vi "db_link.vi"(2 "Current time":timestamp, 4 "SaveNow":bool, 6 "Continuosly":bool, 7 "SaveCurves?":bool, 8 "error in":errorcluster, 9 "AllMeasures":cluster{"x0":dbl, "dx":dbl, "y":sgl[][]}[](array[cluster]), 10 "Table":string[][](array[string]), 11 "reference":refnum<vi>) -> (0 "error":errorcluster)   [LabVIEW 2010]
uses:
  70user.lib/TheSigTab.vi
  <vilib>/addons/database/NI_Database_API.lvlib
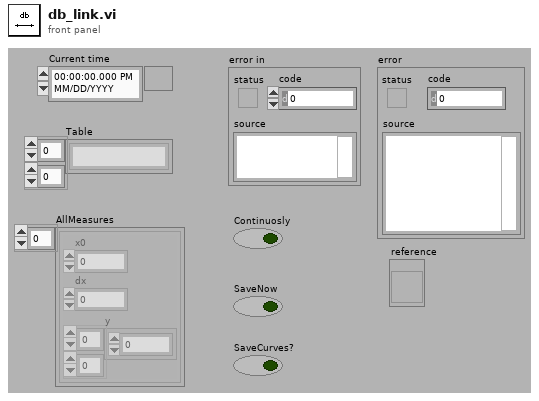
[diagram p1: front panel]
types:
  T1 = typedef "NI_Database_API.lvlib/Conn ObjectReference.ctl" = refnum<k1>
  T2 = cluster{"date/time string":string, "Reason 2":string}
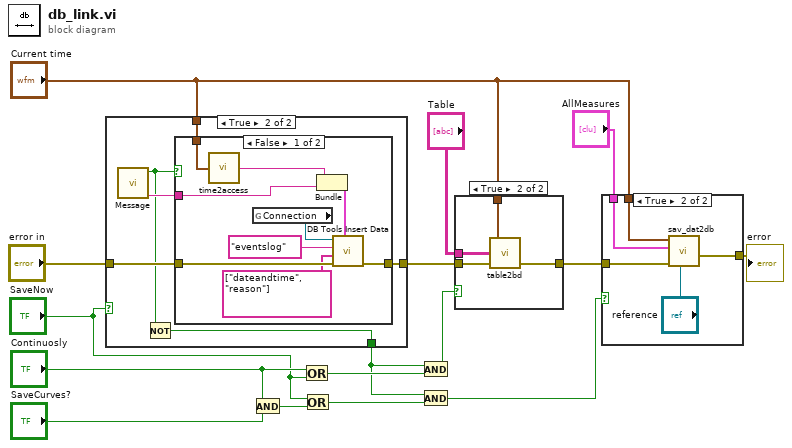
[diagram p0: block diagram]
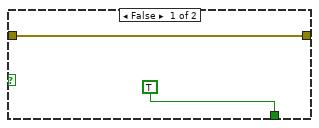
[diagram p4: hidden frame]
diagram:
  n1 = case shown="True" "SaveNow" {
    tunnel: "error in" -> [w18 w23]
    tunnel: "Current time" -> [_ w22]
    tunnel: [w18 w21] -> w14
    tunnel: [TRUE w19] -> w1
    frame False {
    }
    frame True {
      n2 = call "Message.vi"() -> ("Reason 2"=w24:string, "Cancelled?"=w20:bool)  [unwired: 10 in]
      n3 = Not(x=w20) -> (.not. x?=w19:bool)
      n4 = case shown="False" w20 {
        tunnel: [w33 w34] -> w21
        tunnel: w24 -> [w30 _]
        tunnel: w23 -> [w31 w34]
        tunnel: w22 -> [w26 _]
        frame False {
          n5 = call "time2access.vi"("time stamp"=w26) -> ("date/time string"=w25:string)
          n6 = global read "TheSigTab.vi" "Connection"() -> (w28:T1)
          n7 = Bundle("date/time string"=w25, "Reason 2"=w30) -> (w32:T2)  [unwired: 1 in]
          n8 = call <vilib>:"DB Tools Insert Data.vi"("data"=w32, "error in (no error)"=w31, "columns"=string[] ["dateandtime", "reason"], "table"="eventslog", "connection reference"=w28) -> ("error out"=w33:errorcluster)  [unwired: 5 in, 1 out]
        }
        frame True {
        }
      }
    }
  }
  n9 = And(x="Continuosly", y="SaveCurves?") -> (x .and. y?=w7:bool)
  n10 = Or(x="Continuosly", y="SaveNow") -> (x .or. y?=w4:bool)
  n11 = Or(x="SaveNow", y=w7) -> (x .or. y?=w5:bool)
  n12 = And(x=w1, y=w4) -> (x .and. y?=w3:bool)
  n13 = And(x=w1, y=w5) -> (x .and. y?=w2:bool)
  n14 = case shown="True" w3 {
    tunnel: "Table" -> [_ w39]
    tunnel: "Current time" -> [_ w38]
    tunnel: w14 -> [w35 w37]
    tunnel: [w35 w36] -> w12
    frame False {
    }
    frame True {
      n15 = call "table2bd.vi"("error in (no error)"=w37, "eeert"=w39, "time stamp"=w38) -> ("error out"=w36:errorcluster)  [unwired: 2 in]
    }
  }
  n16 = case shown="True" w2 {
    tunnel: "AllMeasures" -> [_ w45]
    tunnel: w12 -> [w40 w44]
    tunnel: [w40 w42] -> w11
    tunnel: "Current time" -> [_ w41]
    frame False {
    }
    frame True {
      n17 = call "sav_dat2db.vi"("Slide Ref"="reference", "error in"=w44, "Array"=w45, "date/time"=w41) -> ("error out"=w42:errorcluster)  [unwired: 5 in]
    }
  }
  "error" <- w11
